vi "Test Deserializations.vi"() -> ()   [LabVIEW 2012]
uses:
  Reusable/PAS/Main/PAS.lvclass
  CRDS/cCRDS/cCRDS.lvclass
panel:
  out "error string":string
  out "error out":errorcluster
  in  "Boolean":bool
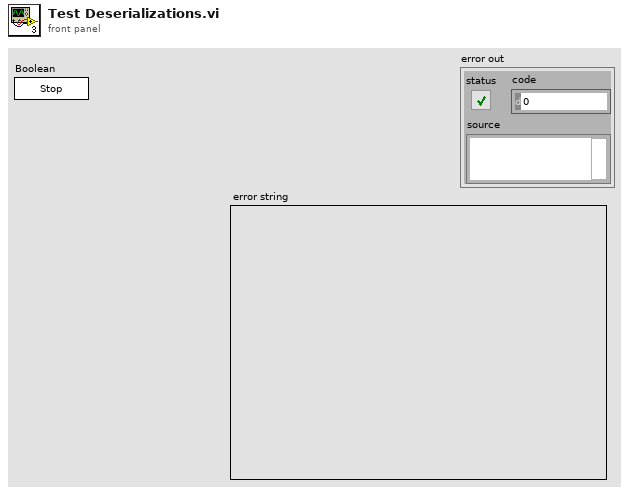
[diagram p1: front panel]
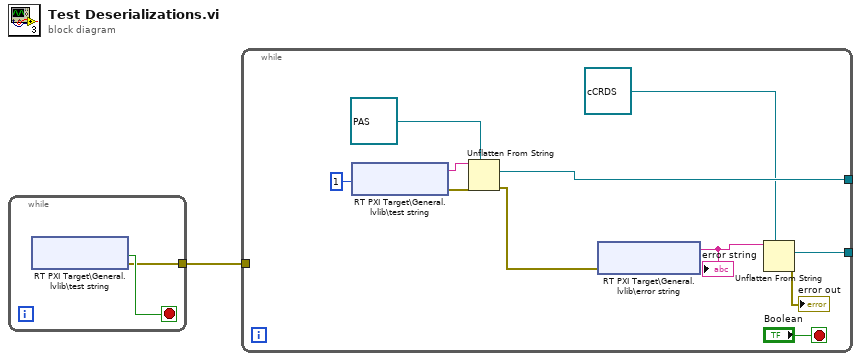
[diagram p0: block diagram]
diagram:
  n1 = while {
    tunnel: [w2] -> w1
    stop <- w3 stop-if-true
    n2 = shared-variable "RT PXI Target\\General.lvlib\\test string"() -> (error out=w2:errorcluster, w3:bool)  [unwired: 2 in, 1 out]
  }
  n3 = while {
    tunnel: w1 -> [_]
    tunnel: [w10] -> _
    tunnel: [w5] -> _
    stop <- "Boolean" stop-if-true
    n4 = shared-variable "RT PXI Target\\General.lvlib\\test string"(1 ("ms timeout (0)")) -> (w12:string, error out=w9:errorcluster)  [unwired: 1 in, 1 out]
    n5 = Unflatten From String(type=refnum<class "PAS.lvclass"> refnum ("PAS"), binary string=w12, error in (no error)=w9) -> (value=w10:refnum<class "PAS.lvclass">, error out=w8:errorcluster)  [unwired: 2 in, 1 out]
    n6 = shared-variable "RT PXI Target\\General.lvlib\\error string"(error in=w8) -> (w7:string)  [unwired: 1 in, 2 out]
    "error string" <- w7
    n7 = Unflatten From String(type=refnum<class "cCRDS.lvclass"> refnum ("cCRDS"), binary string=w7) -> (value=w5:refnum<class "cCRDS.lvclass">, error out=→"error out":errorcluster)  [unwired: 3 in, 1 out]
  }
